vi "Write buffer (as ByteArray).vi"(8 "error in (no error)":errorcluster, 10 "bytes":u8[](array[numeric]) format="%02x", 11 "httpRequest in":refnum<class "httpRequest.lvclass">) -> (0 "error out":errorcluster, 3 "httpRequest out":refnum<class "httpRequest.lvclass">)   [LabVIEW 2020, in "httpClient.lvlib" / "httpRequest.lvclass"]
uses:
  httpRequest.lvclass
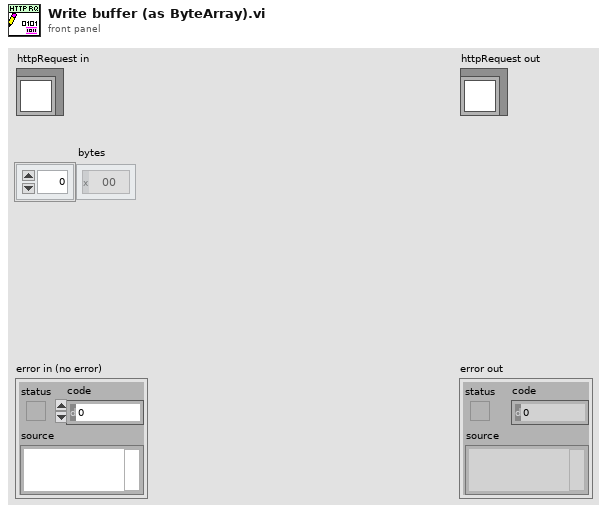
[diagram p1: front panel]
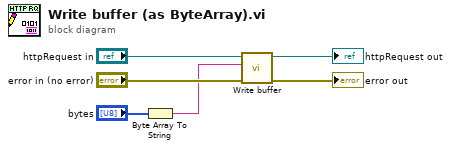
[diagram p0: block diagram]
diagram:
  n1 = Byte Array To String(unsigned byte array="bytes") -> (string=w1:string)
  n2 = call "Write buffer.vi"("error in (no error)"="error in (no error)", "buffer"=w1, "httpRequest in"="httpRequest in") -> ("error out"=→"error out":errorcluster, "httpRequest out"=→"httpRequest out":refnum<class "httpRequest.lvclass">)  [unwired: 7 in]
